vi "init server.vi"(8 "error in (no error)":errorcluster, 11 "Header content in":refnum<class "Header content.lvclass">) -> (0 "error out":errorcluster, 3 "Header content out":refnum<class "Header content.lvclass">)   [LabVIEW 2018, in "Header content.lvclass"]
uses:
  Header content.lvclass
  Server/Server.lvclass
panel:
  in  "Server.lvclass":refnum<class "Server.lvclass">
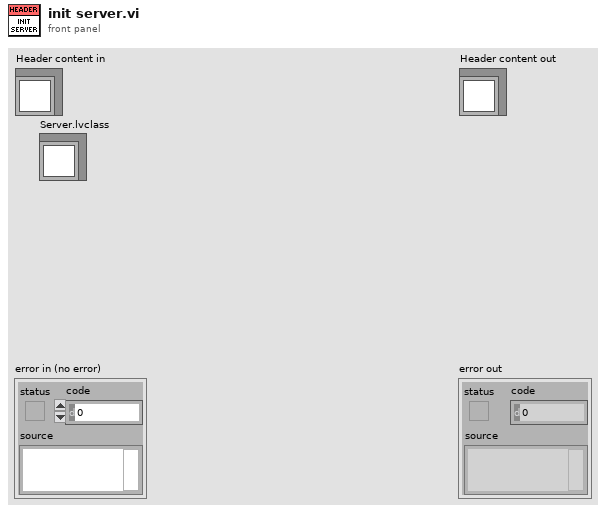
[diagram p1: front panel]
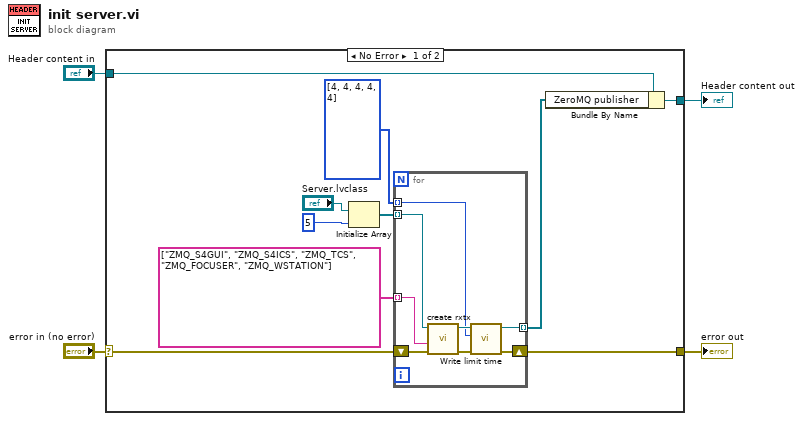
[diagram p0: block diagram]
diagram:
  n1 = case shown="No Error" "error in (no error)" {
    selector: "error in (no error)" -> [w8 w24]
    tunnel: [w14 w24] -> w3
    tunnel: [w13 w23] -> w1
    tunnel: "Header content in" -> [w6 w23]
    frame No Error {
      n2 = Initialize Array("Server.lvclass", 5 ("dimension size")) -> (w12:refnum<class "Server.lvclass">[])
      n3 = for {
        shift-right: [w15] -> w14
        shift-left: w8 -> [w22]
        tunnel: w12 -> [w20] mode=indexing
        tunnel: [w16] -> w10 mode=indexing
        tunnel: string[] ["ZMQ_S4GUI", "ZMQ_S4ICS", "ZMQ_TCS", "ZMQ_FOCUSER", "ZMQ_WSTATION"] -> [w18] mode=indexing
        tunnel: u16[] [4, 4, 4, 4, 4] -> [w17] mode=indexing
        n4 = call "create rxtx.vi"("error in (no error)"=w22, 9:w18, "Server in"=w20) -> ("error out"=w21:errorcluster, "Server out"=w19:refnum<class "Server.lvclass">)  [unwired: 7 in]
        n5 = call "Write limit time.vi"("error in (no error)"=w21, "limit time"=w17, "Server in"=w19) -> ("error out"=w15:errorcluster, "Server out"=w16:refnum<class "Server.lvclass">)  [unwired: 7 in]
      }
      n6 = Bundle By Name(cluster=w6, "ZeroMQ publisher"=w10) -> (w13:refnum<class "Header content.lvclass">)
    }
    frame Error {
    }
  }
  "error out" <- w3
  "Header content out" <- w1
